vi "Solve1.vi"(8 "Error In":errorcluster, 11 "reference in":refnum<class "PuzzleBase.lvclass">) -> (0 "Error Out":errorcluster, 2 "Result":u64, 3 "reference out":refnum<class "PuzzleBase.lvclass">)   [LabVIEW 2020, in "PuzzleBase.lvclass"]
uses:
  PuzzleBase.lvclass
  PuzzleBase.lvclass/PuzzleBase.ctl
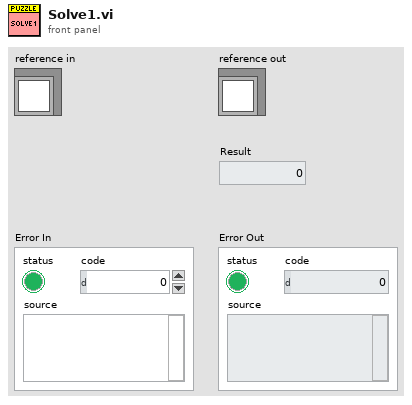
[diagram p1: front panel]
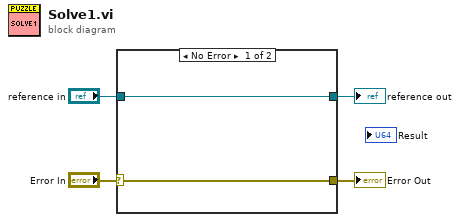
[diagram p0: block diagram]
diagram:
  n1 = case shown="No Error" "Error In" {
    selector: "Error In" -> [w5 w8]
    tunnel: [w5 w8] -> w3
    tunnel: [w6 w7] -> w1
    tunnel: "reference in" -> [w6 w7]
    frame No Error {
    }
    frame Error {
    }
  }
  "Error Out" <- w3
  "reference out" <- w1
